vi "Read Delta.vi"(8 "error in (no error)":errorcluster, 11 "Analyze Results Beam Deviation in":refnum<class "Analyze Results Beam Deviation.lvclass">) -> (0 "error out":errorcluster, 2 "Delta":cluster{"x":sgl, "y":sgl}, 3 "Analyze Results Beam Deviation out":refnum<class "Analyze Results Beam Deviation.lvclass">)   [LabVIEW 2014, in "Analyze Results Beam Deviation.lvclass"]
uses:
  Analyze Results Beam Deviation.lvclass
  Analyze Results Beam Deviation.lvclass/Analyze Results Beam Deviation.ctl
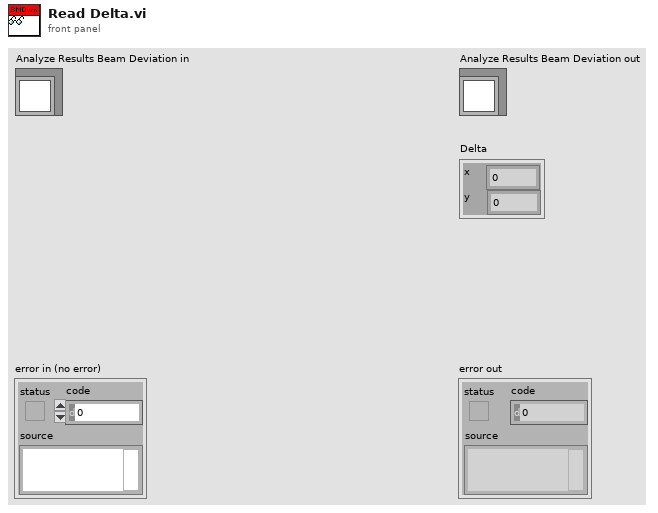
[diagram p1: front panel]
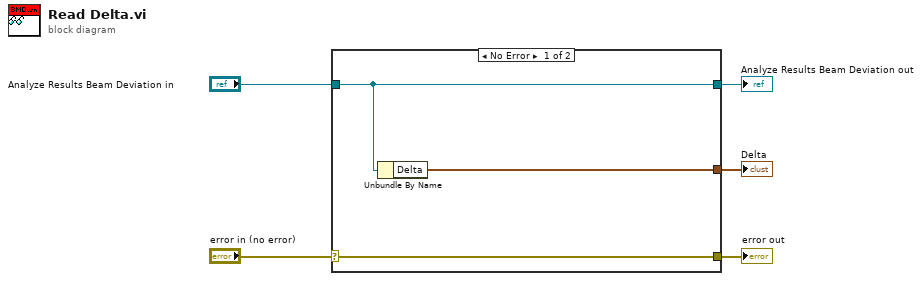
[diagram p0: block diagram]
diagram:
  n1 = case shown="No Error" "error in (no error)" {
    selector: "error in (no error)" -> [w8 w9]
    tunnel: [w8 w9] -> w4
    tunnel: [w7 w10] -> w2
    tunnel: "Analyze Results Beam Deviation in" -> [w7 w10]
    tunnel: [w6 _] -> w1
    frame No Error {
      n2 = Unbundle By Name(w7) -> ("Delta"=w6:cluster{"x":dbl, "y":dbl})
    }
    frame Error {
    }
  }
  "error out" <- w4
  "Analyze Results Beam Deviation out" <- w2
  "Delta" <- w1
